vi "ConfigureMotorType.vi"(0 "axis in":cluster{"keyHandle":u32, "nodeId":u16}={"keyHandle"=0, "nodeId"=1}, 5 "motor type":u16(ring)=10 items=["DC motor"=1, "EC motor (sinus commutated)"=10, "EC motor (block commutated)"=11], 7 "EC motor parameter":T2, 9 "DC motor parameter":T1, 11 "error in (no error)":errorcluster) -> (4 "axis out":cluster{"keyHandle":u32, "nodeId":u16}={"keyHandle"=0, "nodeId"=1}, 15 "error out":errorcluster)   [LabVIEW 2019, in "maxonEPOS.lvlib"]
doc: "<B>ConfigureMotorType</B> writes the correct motor type to the device. Parameters from the motor type can be set."
uses:
  Examples/maxonEPOS.lvlib
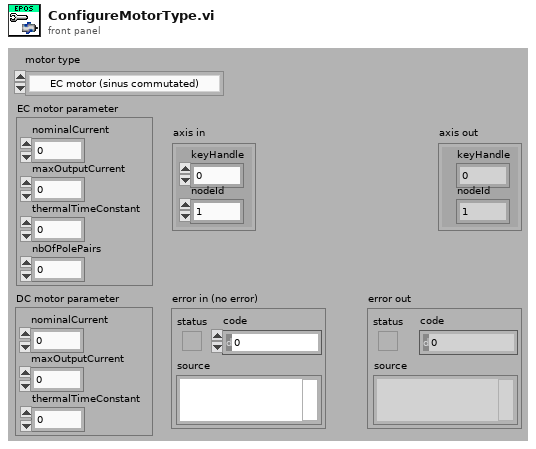
[diagram p1: front panel]
types:
  T1 = cluster{"nominalCurrent":u16, "maxOutputCurrent":u16, "thermalTimeConstant":u16}
  T2 = cluster{"nominalCurrent":u16, "maxOutputCurrent":u16, "thermalTimeConstant":u16, "nbOfPolePairs":u8}
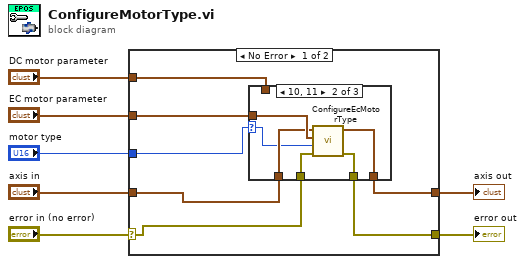
[diagram p0: block diagram]
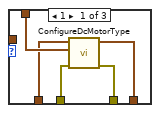
[diagram p2: hidden frame]
diagram:
  n1 = case shown="No Error" "error in (no error)" {
    selector: "error in (no error)" -> [w9 w29]
    tunnel: [w11 w29] -> w6
    tunnel: [w12 w28] -> w5
    tunnel: "axis in" -> [w8 w28]
    tunnel: "motor type" -> [w14 _]
    tunnel: "EC motor parameter" -> [w13 _]
    tunnel: "DC motor parameter" -> [w10 _]
    frame No Error {
      n2 = case shown="10, 11" w14 {
        selector: w14 -> [_ w20 _]
        tunnel: w13 -> [_ w24 _]
        tunnel: w8 -> [w15 w22 w27]
        tunnel: w9 -> [w18 w23 w26]
        tunnel: [w16 w21 w27] -> w12
        tunnel: [w17 w25 w26] -> w11
        tunnel: w10 -> [w19 _ _]
        frame 1 {
          n3 = call "ConfigureDcMotorType.vi"("error in (no error)"=w18, "DC motor parameter"=w19, "axis in"=w15) -> ("error out"=w17:errorcluster, "axis out"=w16:cluster{"keyHandle":u32, "nodeId":u16})  [unwired: 3 in]
        }
        frame 10, 11 {
          n4 = call "ConfigureEcMotorType.vi"("error in (no error)"=w23, "motor type"=w20, "EC motor parameter"=w24, "axis in"=w22) -> ("error out"=w25:errorcluster, "axis out"=w21:cluster{"keyHandle":u32, "nodeId":u16})  [unwired: 2 in]
        }
        frame Default {
        }
      }
    }
    frame Error {
    }
  }
  "error out" <- w6
  "axis out" <- w5
